vi "CRYPrompt Message.vi"() -> (3 "Out":bool)   [LabVIEW 2013]
panel:
  in  "OK":bool
  in  "Prompt":bool caption="aaaa"
  in  "Message":string
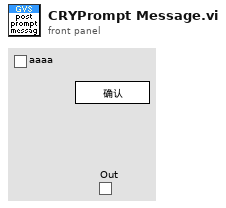
[diagram p1: front panel]
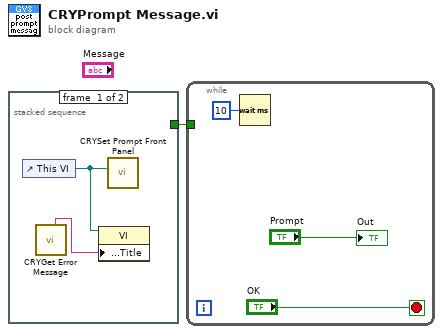
[diagram p0: block diagram]
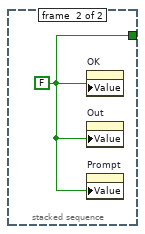
[diagram p2: hidden frame]
diagram:
  n1 = stacked-sequence {
    tunnel: [_ w4] -> w1
    frame #0 {
      n2 = control-ref of="This VI"() -> (w3:refnum<vi>)
      n3 = call "CRYGet Error Message.vi"() -> ("Window Title"=w2:string)  [unwired: 6 in, 5 out]
      n4 = property class="VI"(reference=w3, "Front Panel.Title"=w2) -> ()  [unwired: 1 in, 2 out]
      n5 = call "CRYSet Prompt Front Panel.vi"("Vi Ref"=w3) -> ()  [unwired: 11 in]
    }
    frame #1 {
      w4 = FALSE ("On")
      n6 = property on="OK" class="Bool (strict)"("Value"=w4) -> ()  [unwired: 2 in, 2 out]
      n7 = property on="Out" class="Bool (strict)"("Value"=w4) -> ()  [unwired: 2 in, 2 out]
      n8 = property on="Prompt" class="Bool (strict)"("Value"=w4) -> ()  [unwired: 2 in, 2 out]
    }
  }
  n9 = while {
    tunnel: w1 -> [_]
    stop <- "OK" stop-if-true
    n10 = Wait (ms)(milliseconds to wait=u32 10) -> ()  [unwired: 1 out]
    "Out" <- "Prompt"
  }
